vi "LV SCISDK Get Register.vi"(8 "error in (no error)":errorcluster, 10 "handle":u64, 11 "Path":string) -> (0 "error out":errorcluster, 1 "function return":i32, 2 "handle out":u64, 3 "value":u32)   [LabVIEW 2021, in "SciSDK_Labview.lvlib"]
doc: "SCISDKLABVIEW_DLL_API int LV_SCISDK_GetParameterUInteger(char* Path, unsigned int* value, void* handle);"
uses:
  SciSDK_Labview.lvlib
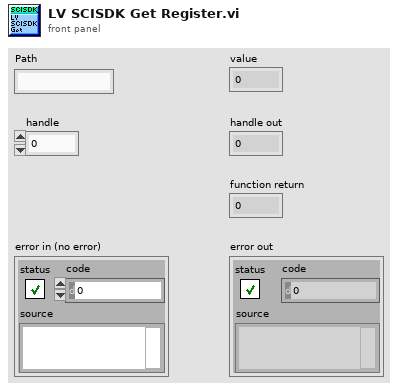
[diagram p1: front panel]
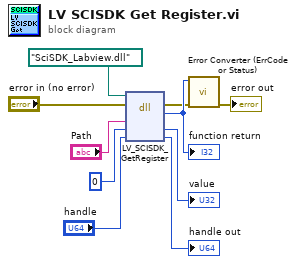
[diagram p0: block diagram]
diagram:
  n1 = dll-call lib="C:/git/scisdk/bin/x64/Release/SciSDK_Labview.dll" fn="LV_SCISDK_GetRegister"(path in=path "SciSDK_Labview.dll", error in="error in (no error)", "Path"="Path", "value"=u32 0, "handle"="handle") -> (error out=w3:errorcluster, "return type"=w10:i32, "value"=→"value":u32, "handle"=→"handle out":u64)  [unwired: 2 in, 1 out]
  "function return" <- w10
  n2 = call <userlib>:"Error Converter (ErrCode or Status).vi"("error in (no error)"=w3, "error code"=w10) -> ("error out"=→"error out":errorcluster)  [unwired: 9 in]
